vi "Is Running.vi"(0 "Engine":refnum<k7>) -> (1 "Running":bool, 2 "Error Out":errorcluster)   [LabVIEW 2021, in "Seq Edit Quick Drop.lvlib"]
uses:
  Seq Edit Quick Drop.lvlib
  Message.ctl
  Command.ctl
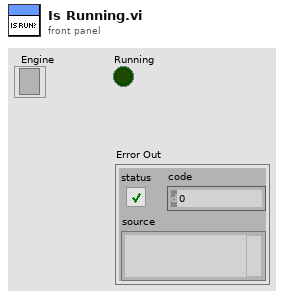
[diagram p1: front panel]
types:
  T1 = typedef "Seq Edit Quick Drop.lvlib/Message.ctl" = cluster{"cmd":T2, "data":variant}
  T2 = typedef "Seq Edit Quick Drop.lvlib/Command.ctl" = enum16{"Init", "Get Application Manager", "Shortcut Activated", "Display Tools", "Tool Selected", "Timeout", "Error", "Close"}
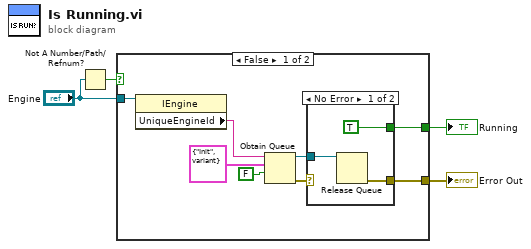
[diagram p0: block diagram]
diagram:
  n1 = Not A Number/Path/Refnum?(number/path/refnum="Engine") -> (NaN/Path/Refnum?=w3:bool)
  n2 = case shown="False" w3 {
    tunnel: "Engine" -> [w12 _]
    tunnel: [w7 _] -> w2
    tunnel: [w6 _] -> w1
    frame False {
      n3 = property class="IEngine"(reference=w12) -> ("UniqueEngineId"=w5:string)  [unwired: 1 in, 2 out]
      n4 = Obtain Queue(name (unnamed)=w5, element data type=T1 {"cmd"=enum."Init", "data"=variant} ("msg"), create if not found? (T)=FALSE) -> (queue out=w9:refnum<queue>, error out=w8:errorcluster)  [unwired: 2 in, 1 out]
      n5 = case shown="No Error" w8 {
        selector: w8 -> [_ w16]
        tunnel: w9 -> [w15 _]
        tunnel: [w14 w16] -> w7
        tunnel: [TRUE _] -> w6
        frame No Error {
          n6 = Release Queue(queue=w15) -> (error out=w14:errorcluster)  [unwired: 2 in, 2 out]
        }
        frame Error {
        }
      }
    }
    frame True {
    }
  }
  "Error Out" <- w2
  "Running" <- w1
